vi "Test Initial Verify.vi"(11 "Test Case In":refnum<class "Basic Mechanics Tests.lvclass">) -> (0 "error out":errorcluster, 3 "Test Case Out":refnum<class "Basic Mechanics Tests.lvclass">)   [LabVIEW 2020, in "Basic Mechanics Tests.lvclass"]
uses:
  Basic Mechanics Tests.lvclass
  C:/Program Files/National Instruments/LabVIEW 2026/vi.lib/Astemes/LUnit/Test Case.lvclass
  Source/Approval Tests/Options/Options.lvclass
  Source/Approval Tests/Report Nothing/Report Nothing.lvclass
  C:/Users/SAS/Desktop/ApprovalTests.LabVIEW/Source/Approval Tests/Reporter/Reporter.lvclass
  <vilib>/Astemes/LUnit/Test Case.lvclass/Test Case.ctl
  Source/Approval Tests/Options/Options.lvclass/Options.ctl
  Source/Approval Tests/Naming Data/Naming Data.lvclass/Naming Data.ctl
  4be351cf-9afa-44a9-9686-c31d6937e1da.vi
  5b6af433-73f2-478c-ac60-49e9a84e5db2.vi
  fbf3a6f1-25d3-4b1a-9ed1-fe282719be7b.vi
  Source/Approval Tests/Options/Write Reporter.vi
  <vilib>/Astemes/LUnit/Core/LUnit Test Case/Private/Append Pass Result.vi
  <vilib>/Astemes/LUnit/Core/LUnit Test Case/Private/Append Fail Result.vi
  Source/Approval Tests/Verify Core.vi
  4be351cf-9afa-44a9-9686-c31d6937e1da.vi/93c5622b-9fb7-41e0-8c76-3fde37e94e34.vi
  Source/Approval Tests/Options/Update Test Name if Not Defined.vi
  Source/Approval Tests/Options/Read Scrubber.vi
  5b6af433-73f2-478c-ac60-49e9a84e5db2.vi/9c5d11cd-9439-4240-a1ee-d9baace9c924.vi
  fbf3a6f1-25d3-4b1a-9ed1-fe282719be7b.vi/9c5d11cd-9439-4240-a1ee-d9baace9c924.vi
  <vilib>/Astemes/LUnit/Core/LUnit Test Case/Private/Run In UI.vi
  Source/Approval Tests/Options/Read Namer.vi
  Source/Approval Tests/Options/Read Naming Data.vi
  Source/Approval Tests/Options/Read Reporter.vi
  Source/Approval Tests/Options/Read Text Comparator.vi
  4be351cf-9afa-44a9-9686-c31d6937e1da.vi/93c5622b-9fb7-41e0-8c76-3fde37e94e34.vi/04cb982b-2eda-40d0-8d7e-90f8e0b569b2.vi
  Source/Approval Tests/Naming Data/Read Test VI Name.vi
  Source/Approval Tests/Naming Data/Write Test VI Name.vi
  Source/Approval Tests/Options/Add Label to Namer.vi
  Source/Approval Tests/conv EOL.vi
  Source/Approval Tests/Reporter/Report.vi
  Source/Approval Tests/Scrubber/Scrubber.lvclass
  Source/Approval Tests/Namer/Namer.lvclass
  Source/Approval Tests/Naming Data/Naming Data.lvclass
  Source/Approval Tests/Reporter/Reporter.lvclass
  Source/Approval Tests/Text Comparator/Text Comparator.lvclass
  <vilib>/Astemes/LUnit/Test Case.lvclass
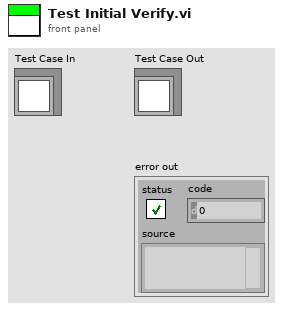
[diagram p1: front panel]
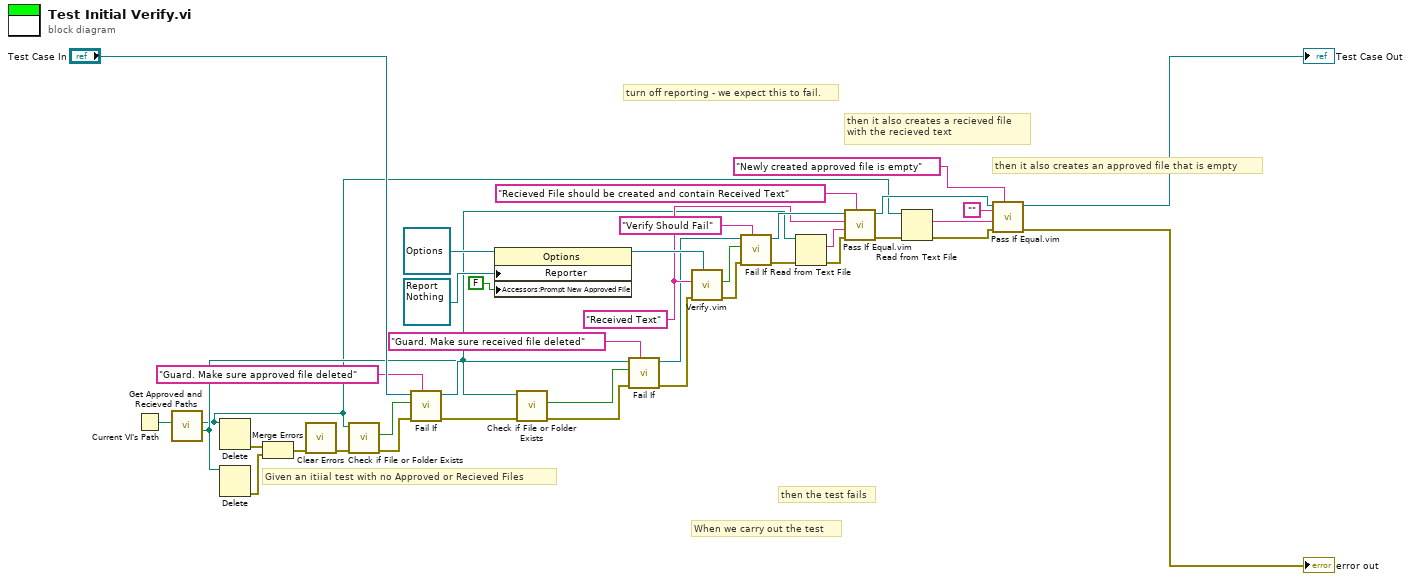
[diagram p0: block diagram]
diagram:
  w20 = "Received Text"
  # "then it also creates an approved file that is empty"
  # "then it also creates a recieved file\nwith the recieved text"
  # "then the test fails"
  # "When we carry out the test"
  # "Given an itiial test with no Approved or Recieved Files"
  # "turn off reporting - we expect this to fail."
  n1 = Current VI's Path() -> (path=w15:path)
  n2 = call "Get Approved and Recieved Paths.vi"("This VI"=w15) -> ("Recieved"=w5:path, "Approved Path"=w2:path)  [unwired: 9 in]
  n3 = Delete(path (use dialog)=w2) -> (error out=w33:errorcluster)  [unwired: 4 in, 2 out]
  n4 = Delete(path (use dialog)=w5) -> (error out=w32:errorcluster)  [unwired: 4 in, 2 out]
  n5 = Merge Errors(w33, w32) -> (w27:errorcluster)
  n6 = call <vilib>:"Clear Errors.vi"("error in (no error)"=w27) -> ("error out"=w26:errorcluster)  [unwired: 5 in, 1 out]
  n7 = call <vilib>:"Check if File or Folder Exists.vi"("error in (no error)"=w26, "path"=w2) -> ("error out"=w29:errorcluster, "file or folder exists?"=w7:bool)  [unwired: 7 in, 1 out]
  n8 = call <vilib>:"Fail If.vi"("Description"="Guard. Make sure approved file deleted", "error in (no error)"=w29, "Fail?"=w7, "LUnit Test Case In"="Test Case In") -> ("error out"=w31:errorcluster, "LUnit Test Case Out"=w9:refnum<class "Basic Mechanics Tests.lvclass">)  [unwired: 6 in]
  n9 = property on="Property Node" class="Options"(reference=refnum<class "Options.lvclass"> refnum ("Options"), "Reporter"=refnum<class "Report Nothing.lvclass"> refnum ("Approval Tests.lvlib:Report Nothing"), "Accessors:Prompt New Approved File"=FALSE ("Prompt New Approved File")) -> (reference out=w24:refnum<class "Options.lvclass">)  [unwired: 1 in, 1 out]
  n10 = call <vilib>:"Check if File or Folder Exists.vi"("error in (no error)"=w31, "path"=w5) -> ("error out"=w28:errorcluster, "file or folder exists?"=w4:bool)  [unwired: 7 in, 1 out]
  n11 = call <vilib>:"Fail If.vi"("Description"="Guard. Make sure received file deleted", "error in (no error)"=w28, "Fail?"=w4, "LUnit Test Case In"=w9) -> ("error out"=w30:errorcluster, "LUnit Test Case Out"=w8:refnum<class "Basic Mechanics Tests.lvclass">)  [unwired: 6 in]
  n12 = call "Verify.vim"("Options"=w24, "error in"=w30, "Anything"=w20) -> ("error out"=w36:errorcluster, "Passed?"=w22:bool)  [unwired: 6 in, 1 out]
  n13 = call <vilib>:"Fail If.vi"("Description"="Verify Should Fail", "error in (no error)"=w36, "Fail?"=w22, "LUnit Test Case In"=w8) -> ("error out"=w35:errorcluster, "LUnit Test Case Out"=w21:refnum<class "Basic Mechanics Tests.lvclass">)  [unwired: 6 in]
  n14 = Read from Text File(file (use dialog)=w5, error in=w35) -> (text=w19:string, error out=w34:errorcluster)  [unwired: 2 in, 2 out]
  n15 = call "Pass If Equal.vim"("Description"="Recieved File should be created and contain Received Text", "error in (no error)"=w34, "Actual"=w19, "Expected"=w20, "LUnit Test Case In"=w21) -> ("error out"=w37:errorcluster, "LUnit Test Case Out"=w18:refnum<class "Basic Mechanics Tests.lvclass">)  [unwired: 5 in]
  n16 = Read from Text File(file (use dialog)=w2, error in=w37) -> (text=w16:string, error out=w38:errorcluster)  [unwired: 2 in, 2 out]
  n17 = call "Pass If Equal.vim"("Description"="Newly created approved file is empty", "error in (no error)"=w38, "Actual"=w16, "Expected"="", "LUnit Test Case In"=w18) -> ("error out"=→"error out":errorcluster, "LUnit Test Case Out"=→"Test Case Out":refnum<class "Basic Mechanics Tests.lvclass">)  [unwired: 5 in]
